vi "LDA_meas_global_1.vi"() -> ()   [LabVIEW 2018]
panel:
  in  "LDA Results file Values":string[](array[string])
  in  "LDA Results file headers":string[](array[string])
  in  "Transit times":dbl[](array[numeric]) format="%.2f"
  in  "Arrival times":dbl[](array[numeric]) format="%.2f"
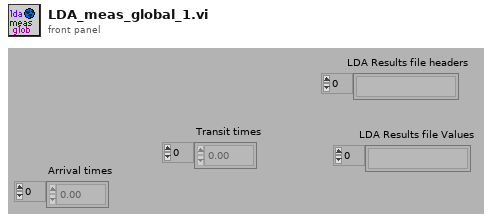
[diagram p1: front panel]
diagram:
